vi "Solution part 2.vi"() -> ()   [LabVIEW 2020]
panel:
  out "result":i16
  in  "data?":bool
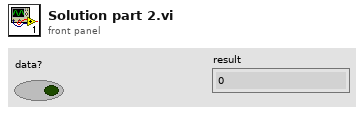
[diagram p1: front panel]
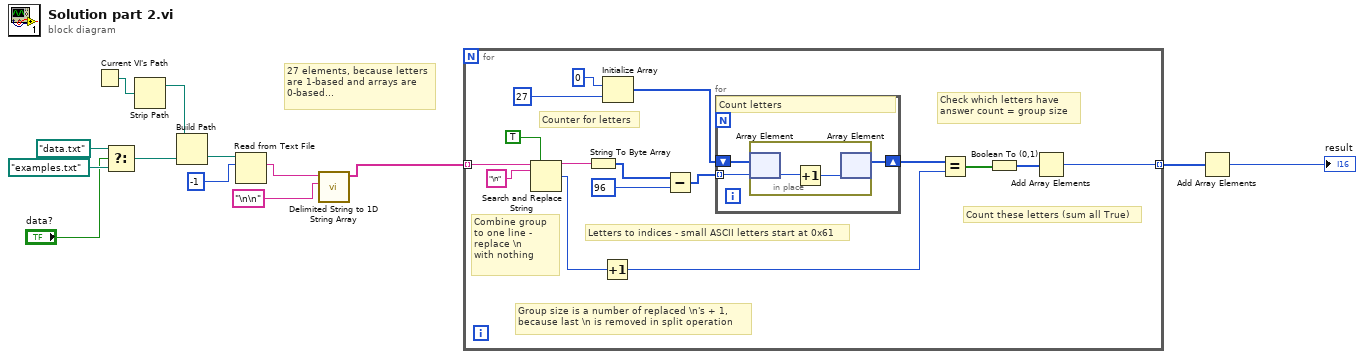
[diagram p0: block diagram]
diagram:
  # "27 elements, because letters\nare 1-based and arrays are\n0-based..."
  n1 = Current VI's Path() -> (path=w9:path)
  n2 = Select(t=path "data.txt", s="data?", f=path "examples.txt") -> (s? t:f=w10:path)
  n3 = Strip Path(path=w9) -> (stripped path=w8:path)  [unwired: 1 out]
  n4 = Build Path(base path=w8, name or relative path=w10) -> (appended path=w7:path)
  n5 = Read from Text File(file (use dialog)=w7, count=-1) -> (text=w4:string)  [unwired: 2 in, 3 out]
  n6 = call <vilib>:"Delimited String to 1D String Array.vi"("delimiter"="\n\n", "delimited string"=w4) -> ("string array"=w3:string[])  [unwired: 9 in]
  n7 = for {
    tunnel: w3 -> [w29] mode=indexing
    tunnel: [w17] -> w1 mode=indexing
    # "Combine group\nto one line - \nreplace \\n\nwith nothing"
    # "Letters to indices - small ASCII letters start at 0x61"
    # "Count these letters (sum all True)"
    # "Check which letters have \nanswer count = group size"
    # "Counter for letters"
    # "Group size is a number of replaced \\n's + 1,\nbecause last \\n is removed in split operation"
    n8 = Search and Replace String(replace all?=TRUE ("replace all? (F)"), input string=w29, search string="\n") -> (result string=w26:string, number of replacements=w23:i32)  [unwired: 5 in, 2 out]
    n9 = String To Byte Array(string=w26) -> (unsigned byte array=w25:u8[])
    n10 = Increment(x=w23) -> (x+1=w20:i32)
    n11 = Initialize Array(0, 27) -> (w14:i32[])
    n12 = Subtract(x=w25, y=u8 96) -> (x-y=w22:u8[])
    n13 = for {
      tunnel: w22 -> [w31] mode=indexing
      shift-right: [w30] -> w21
      shift-left: w14 -> [w32]
      # "Count letters"
      n14 = in-place {
        n15 = in-place-array #1(w32, w31) -> (w34:i32)
        n16 = Increment(x=w34) -> (x+1=w33:i32)
        n17 = in-place-array #1(w33) -> (w30:i32[])  [unwired: 1 out]
      }
    }
    n18 = Equal?(x=w21, y=w20) -> (x = y?=w19:bool[])
    n19 = Boolean To (0,1)(Boolean=w19) -> (0, 1=w18:i16[])
    n20 = Add Array Elements(numeric array=w18) -> (sum=w17:i16)
  }
  n21 = Add Array Elements(numeric array=w1) -> (sum=→"result":i16)
